vi "connect_SLM.vi"(8 "error in (no error)":errorcluster, 11 "Required SDK version":T1={"Major Version Number"=4, "Minor Version Number"=1}) -> (1 "SLM connected":bool, 3 "SLM ID":T2)   [LabVIEW 2025]
uses:
  <userlib>/HOLOEYE SLM Display SDK 4.1.0/types/heds_slm_id_typedef.ctl
  <userlib>/HOLOEYE SLM Display SDK 4.1.0/types/heds_required_sdk_version_typedef.ctl
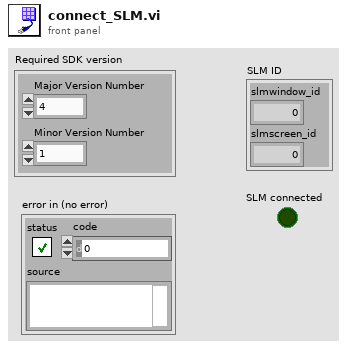
[diagram p1: front panel]
types:
  T1 = typedef "heds_required_sdk_version_typedef.ctl" = cluster{"Major Version Number":i32, "Minor Version Number":i32}
  T2 = typedef "heds_slm_id_typedef.ctl" = cluster{"slmwindow_id":u32, "slmscreen_id":u32}
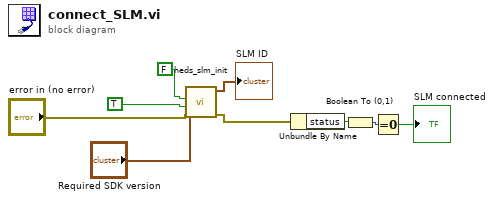
[diagram p0: block diagram]
diagram:
  n1 = call <userlib>:"heds_slm_init.vi"("error in (no error)"="error in (no error)", "Close open SLM windows (T)"=TRUE, "Show Preview (T)"=FALSE, "Required SDK version"="Required SDK version") -> ("error out"=w3:errorcluster, "SLM ID"=→"SLM ID":T2)  [unwired: 6 in]
  n2 = Unbundle By Name(w3) -> ("status"=w5:bool)
  n3 = Boolean To (0,1)(Boolean=w5) -> (0, 1=w6:i16)
  n4 = Equal To 0?(x=w6) -> (x = 0?=→"SLM connected":bool)
